vi "meas_in_pixel.vi"(8 "error in (no error)":errorcluster, 9 "Search Lines":T3[](array[typedef]) {"Edge Info"."Distance (Real-World)" format="%.2f"; "Edge Info"."Location (Real-World)"."Y" format="%.2g"; "Edge Info"."Location (Real-World)"."X" format="%.2f"; "Edge Info"."Noise" format="%.2f"; "Edge Info"."Location (Pixel)"."Y" format="%.2g"; "Edge Info"."Location (Pixel)"."X" format="%.2f"; "Edge Info"."Strength" format="%.2f"; "Edge Info"."Distance (Pixel)" format="%.2f"}, 10 "Last Edges":T4[](array[typedef]) {"Distance (Real-World)" format="%.2f"; "Location (Real-World)"."Y" format="%.2g"; "Location (Real-World)"."X" format="%.2f"; "Noise" format="%.2f"; "Location (Pixel)"."Y" format="%.2g"; "Location (Pixel)"."X" format="%.2f"; "Strength" format="%.2f"; "Distance (Pixel)" format="%.2f"}, 11 "First Edges":T4[](array[typedef]) {"Distance (Real-World)" format="%.2f"; "Location (Real-World)"."Y" format="%.2g"; "Location (Real-World)"."X" format="%.2f"; "Noise" format="%.2f"; "Location (Pixel)"."Y" format="%.2g"; "Location (Pixel)"."X" format="%.2f"; "Strength" format="%.2f"; "Distance (Pixel)" format="%.2f"}) -> (0 "error out":errorcluster, 2 "Points for Arrow Overlay":T1, 3 "Algo Output":T2)   [LabVIEW 2019, in "Algorithm.lvclass"]
uses:
  FrameworkOverrides/Algorithm.lvclass
  <vilib>/vision/NI_Vision_Development_Module.lvlib
  <vilib>/vision/Measure.llb/Edge New.ctl
  <vilib>/vision/Measure.llb/Search Line.ctl
panel:
  out "Array":sgl[](array[numeric])
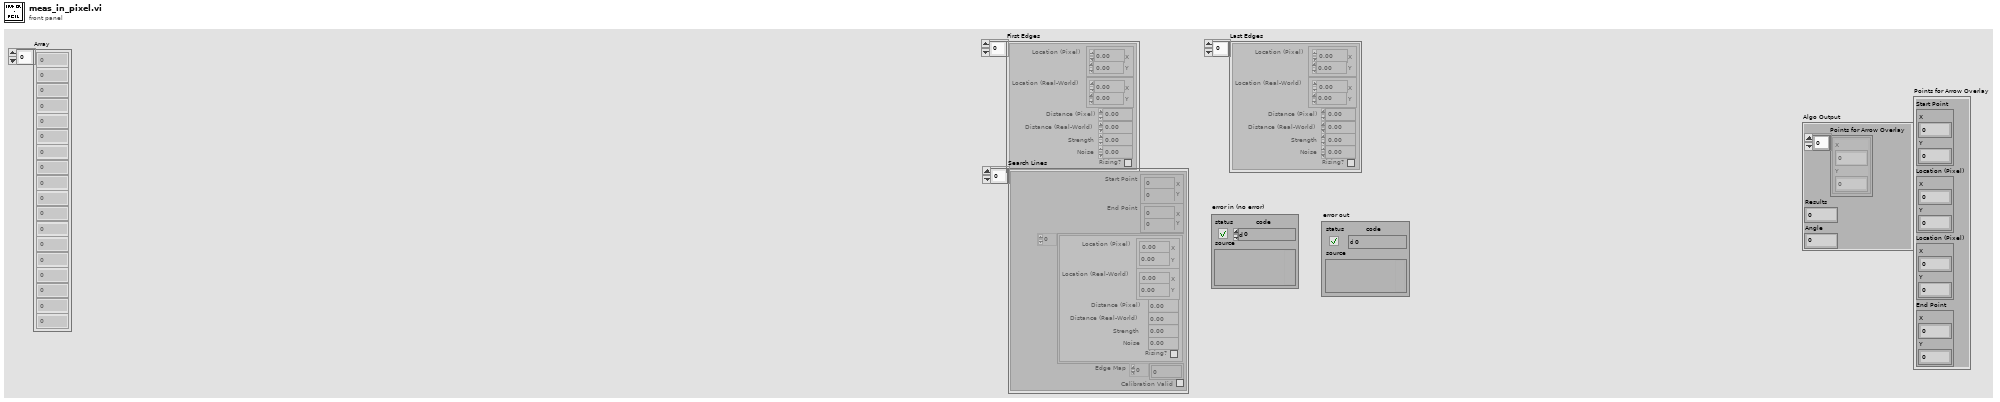
[diagram p1: front panel]
types:
  T1 = cluster{"Start Point":cluster{"X":sgl, "Y":sgl}, "Location (Pixel)":cluster{"X":sgl, "Y":sgl}, "Location (Pixel)":cluster{"X":sgl, "Y":sgl}, "End Point":cluster{"X":sgl, "Y":sgl}}
  T2 = cluster{"Points for Arrow Overlay":cluster{"X":sgl, "Y":sgl}[], "Results":sgl, "Angle":sgl}
  T3 = typedef "Search Line.ctl" = cluster{"Start Point":cluster{"X":sgl, "Y":sgl}, "End Point":cluster{"X":sgl, "Y":sgl}, "Edge Info":T4[], "Edge Map":dbl[], "Calibration Valid":bool}
  T4 = typedef "Edge New.ctl" = cluster{"Location (Pixel)":cluster{"X":sgl, "Y":sgl}, "Location (Real-World)":cluster{"X":sgl, "Y":sgl}, "Distance (Pixel)":dbl, "Distance (Real-World)":dbl, "Strength":dbl, "Noise":dbl, "Rising?":bool}
  T5 = cluster{"Points for Arrow Overlay":cluster{"X":sgl, "Y":sgl}[], "Numeric":sgl, "Angle":sgl}
  T6 = cluster{"Location (Pixel)":cluster{"X":sgl, "Y":sgl}, "Location (Pixel)":cluster{"X":sgl, "Y":sgl}}
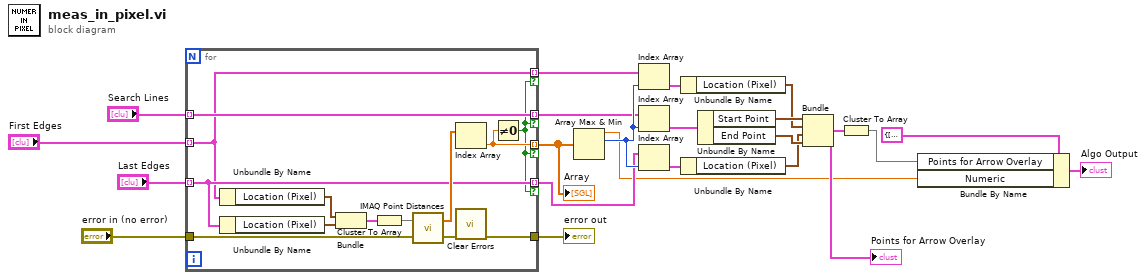
[diagram p0: block diagram]
diagram:
  n1 = for {
    tunnel: "First Edges" -> [w30] mode=indexing
    tunnel: "Last Edges" -> [w31] mode=indexing
    tunnel: "Search Lines" -> [w32] mode=indexing
    tunnel: [w34] -> w7 mode=indexing if=w29
    tunnel: "error in (no error)" -> [w23]
    tunnel: [w25] -> w3
    tunnel: [w32] -> w5 mode=indexing if=w29
    tunnel: [w31] -> w4 mode=indexing if=w29
    tunnel: [w30] -> w6 mode=indexing if=w29
    n2 = Unbundle By Name(w30) -> ("Location (Pixel)"=w28:cluster{"X":sgl, "Y":sgl})
    n3 = Unbundle By Name(w31) -> ("Location (Pixel)"=w27:cluster{"X":sgl, "Y":sgl})
    n4 = Bundle("Location (Pixel)"=w28, "Location (Pixel)"=w27) -> (w33:T6)  [unwired: 1 in]
    n5 = Cluster To Array(cluster=w33) -> (array=w24:cluster{"X":sgl, "Y":sgl}[])
    n6 = call "IMAQ Point Distances"("Points"=w24, "error in (no error)"=w23) -> ("Distances"=w35:sgl[], "error out"=w26:errorcluster)  [unwired: 3 in]
    n7 = Index Array(array=w35) -> (element=w34:sgl)  [unwired: 1 in]
    n8 = call <vilib>:"Clear Errors.vi"("error in (no error)"=w26) -> ("error out"=w25:errorcluster)  [unwired: 5 in, 1 out]
    n9 = Not Equal To 0?(x=w34) -> (x != 0?=w29:bool)
  }
  "Array" <- w7
  "error out" <- w3
  n10 = Array Max & Min(array=w7) -> (max value=w1:sgl, max index (indices)=w14:i32)  [unwired: 2 out]
  n11 = Index Array(array=w6, index=w14) -> (element=w15:T4)
  n12 = Index Array(array=w5, index=w14) -> (element=w12:T3)
  n13 = Index Array(array=w4, index=w14) -> (element=w13:T4)
  n14 = Unbundle By Name(w15) -> ("Location (Pixel)"=w9:cluster{"X":sgl, "Y":sgl})
  n15 = Unbundle By Name(w13) -> ("Location (Pixel)"=w8:cluster{"X":sgl, "Y":sgl})
  n16 = Unbundle By Name(w12) -> ("Start Point"=w11:cluster{"X":sgl, "Y":sgl}, "End Point"=w10:cluster{"X":sgl, "Y":sgl})
  n17 = Bundle("Start Point"=w11, "Location (Pixel)"=w9, "Location (Pixel)"=w8, "End Point"=w10) -> (w2:T1)  [unwired: 1 in]
  "Points for Arrow Overlay" <- w2
  n18 = Cluster To Array(cluster=w2) -> (array=w16:cluster{"X":sgl, "Y":sgl}[])
  n19 = Bundle By Name(cluster=T5 {"Points for Arrow Overlay"=[], "Numeric"=0.0, "Angle"=0.0}, "Points for Arrow Overlay"=w16, "Numeric"=w1) -> (→"Algo Output":T5)
